vi "Test SCOPE API.vi"() -> ()   [LabVIEW 2021, in "SCOPE.lvlib"]
doc: "SCOPE API Tester.\n\n<b>Note:</b> This VI was modified by the <b>Validate DQMH Module</b> tool to add the 'Show Main VI Diagram on Init' functionality included in DQMH 6.1.\n\n<b>Note:</b> This VI was modified by the <b>Validate DQMH Module</b> tool to upgrade its Error Reported event frame to use an improved mechanism for displaying error information.\n\n<b>Note:</b> This VI was modified by the <b>Validate DQMH Module</b> tool to remove code to stop the main loop on error, and instead display the most recent error on the tester front panel."
uses:
  SCOPE.lvlib
  <vilib>/Utility/error.llb/DialogType.ctl
panel:
  in  "UnLoad in SubPane":bool
  in  "Load in SubPane":bool
  out "last error":errorcluster
  in  "Show Main VI Diagram on Init (F)":bool
  in  "AcqTime":dbl=20.0
  in  "Acquire Signal":bool
  out "ModuleName":string
  in  "Sim?":bool
  in  "Simulation":bool
  in  "Show Block Diagram":bool
  in  "Stop Module":bool
  in  "Start Module":bool
  in  "Hide Module Panel":bool
  in  "Show Module Panel":bool
  out "Status":string
  out "Module Running?":bool
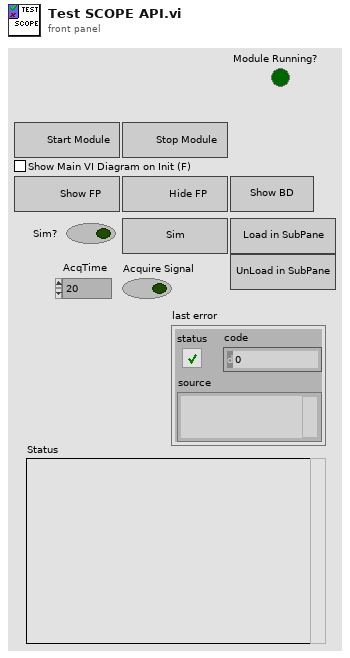
[diagram p1: front panel]
types:
  T1 = typedef "SCOPE.lvlib/Broadcast Events--cluster.ctl" = cluster{"Module Did Init":refnum<user-event>, "Status Updated":refnum<user-event>, "Error Reported":refnum<user-event>, "Module Did Stop":refnum<user-event>, "Update Module Execution Status":refnum<user-event>}
  T2 = typedef "DialogType.ctl" = u16
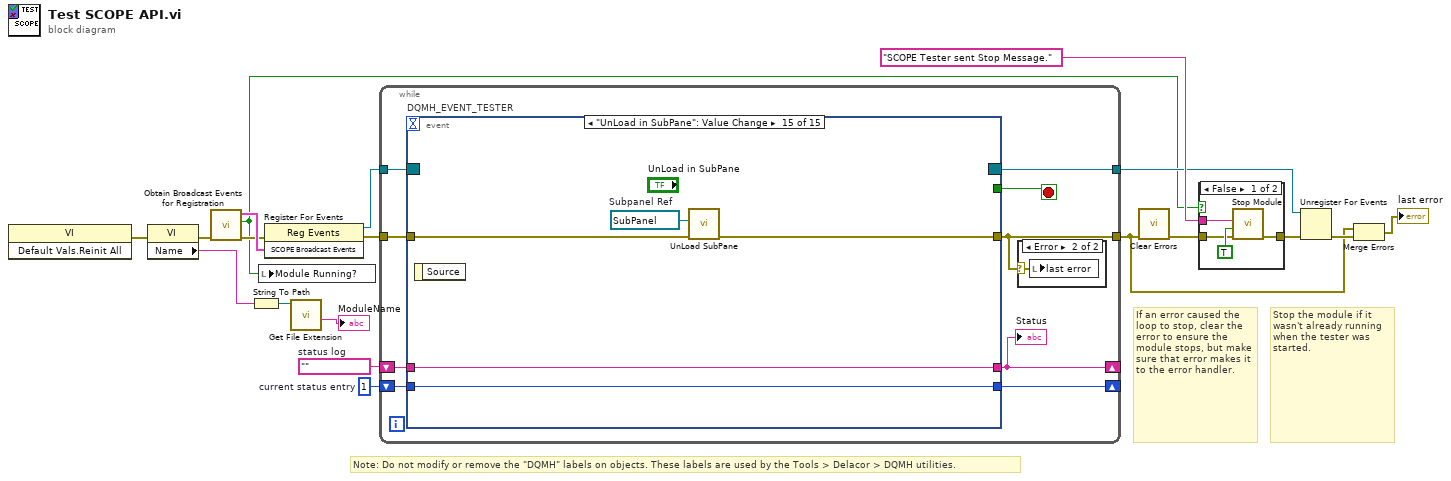
[diagram p0: block diagram]
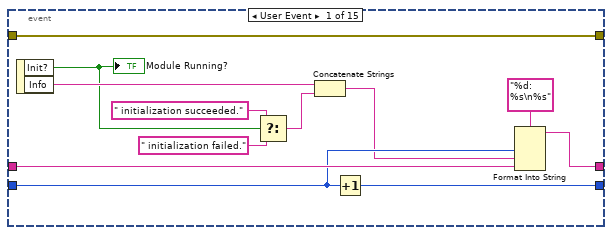
[diagram p4: hidden frame]
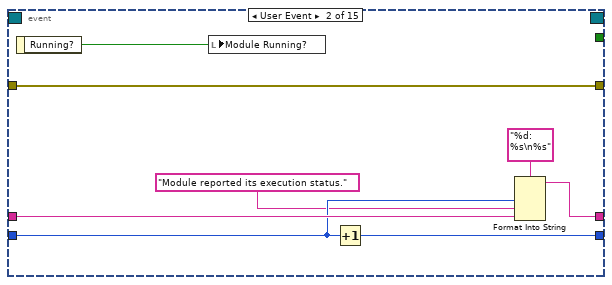
[diagram p5: hidden frame]
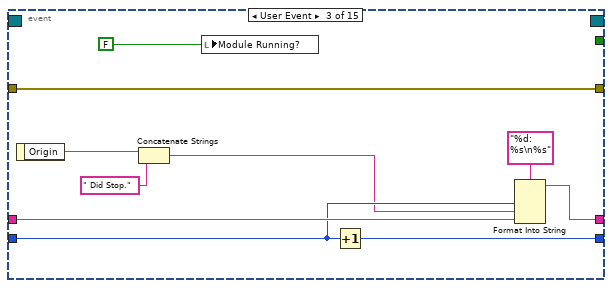
[diagram p6: hidden frame]
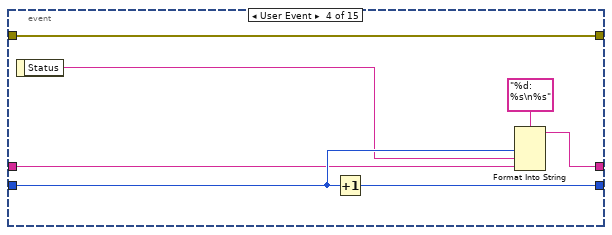
[diagram p7: hidden frame]
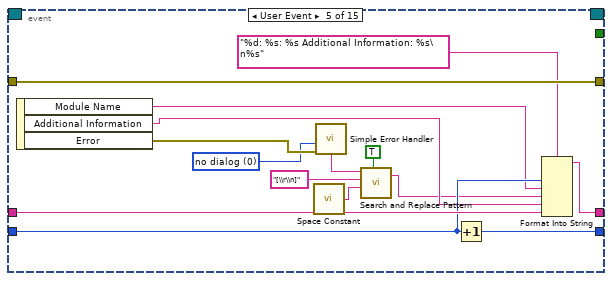
[diagram p8: hidden frame]
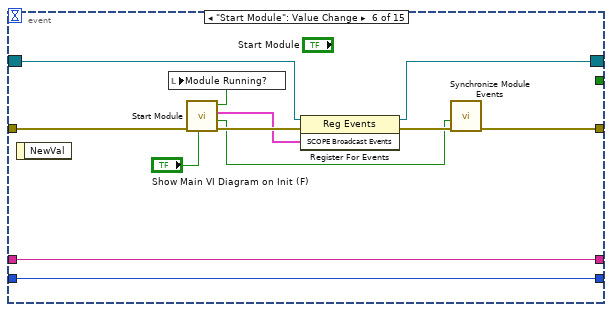
[diagram p9: hidden frame]
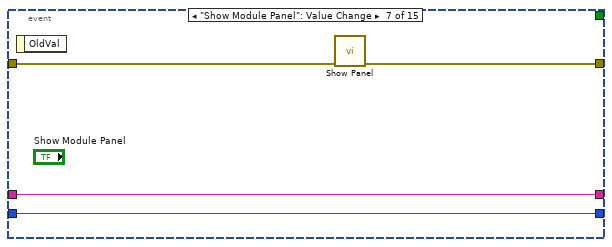
[diagram p10: hidden frame]
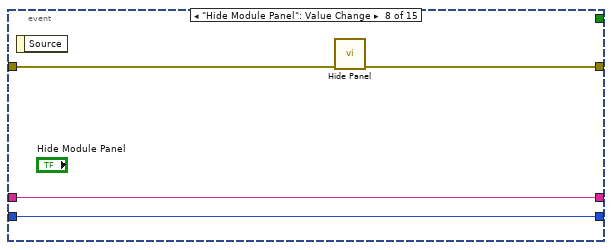
[diagram p11: hidden frame]
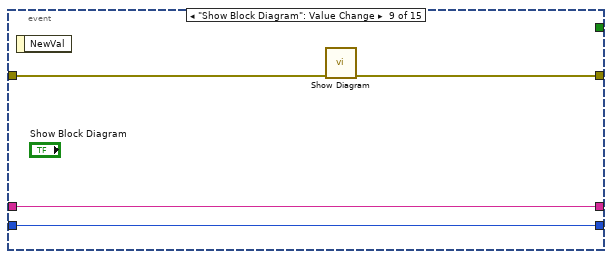
[diagram p12: hidden frame]
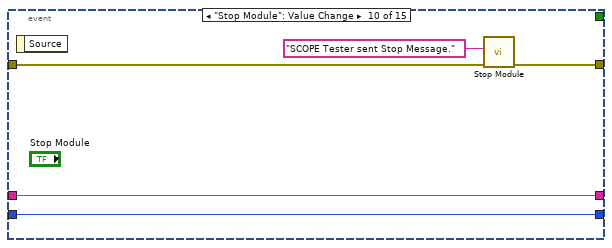
[diagram p13: hidden frame]
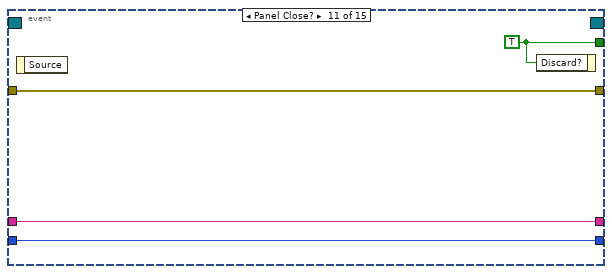
[diagram p14: hidden frame]
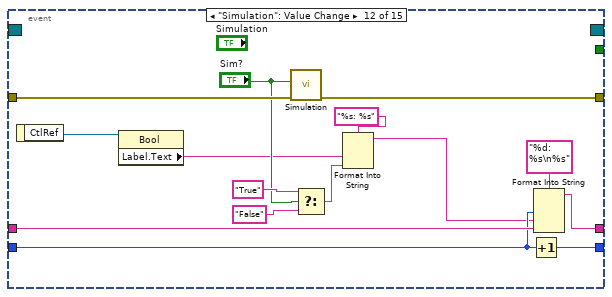
[diagram p15: hidden frame]
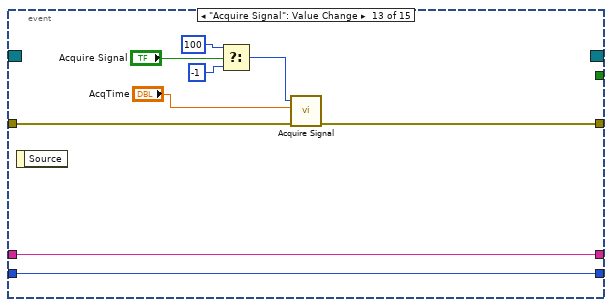
[diagram p16: hidden frame]
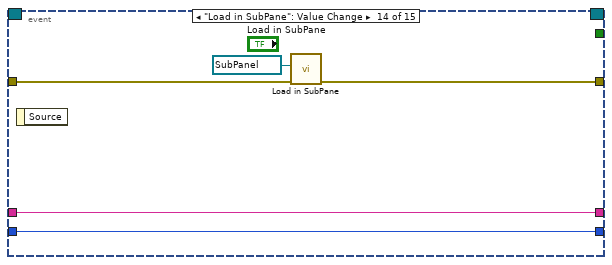
[diagram p17: hidden frame]
diagram:
  w15 = 1  # current status entry
  w16 = ""  # status log
  # "Stop the module if it wasn't already running when the tester was started."
  # "If an error caused the loop to stop, clear the error to ensure the module stops, but make sure that error makes it to the error handler."
  # "Note: Do not modify or remove the \"DQMH\" labels on objects. These labels are used by the Tools > Delacor > DQMH utilities."
  n1 = invoke on="Invoke Node" class="VI" method="Default Vals.Reinit All"() -> (error out=w6:errorcluster)  [unwired: 3 in, 2 out]
  n2 = property on="Property Node" class="VI"(error in=w6) -> (error out=w5:errorcluster, "Name"=w3:string)  [unwired: 1 in, 1 out]
  n3 = call "Obtain Broadcast Events for Registration.vi"("error in (no error)"=w5) -> ("error out"=w8:errorcluster, "Already running?"=w7:bool, "SCOPE Broadcast Events"=w13:T1)  [unwired: 8 in]
  n4 = String To Path(string=w3) -> (path=w2:path)
  n5 = local write "Module Running?"(w7) -> ()
  n6 = register-events(error in=w8, w13) -> (reference out=w12:refnum<event-registration>, error out=w14:errorcluster)  [unwired: 1 in]
  n7 = call <vilib>:"Get File Extension.vi"("file"=w2) -> ("filename without extension"=→"ModuleName":string)  [unwired: 6 in, 4 out]
  n8 = while {
    tunnel: w12 -> [w28]
    tunnel: [w21] -> w9
    shift-right: [w24] -> _
    shift-left: w16 -> [w26]
    shift-right: [w25] -> _
    shift-left: w15 -> [w27]
    tunnel: w14 -> [w23]
    tunnel: [w22] -> w11
    stop <- w20 stop-if-true
    n9 = event "DQMH_EVENT_TESTER" shown="[14] \"UnLoad in SubPane\": Value Change" {
      selector: w28 -> [_ _ _ _ _ w87 _ _ _ _ _ _ _ _ _]
      dyn-events: [_ _ _ _ _ w86 _ _ _ _ _ _ _ _ _] -> w22
      timeout: _ -> [_ _ _ _ _ _ _ _ _ _ _ _ _ _ _]
      tunnel: [_ _ _ _ _ _ _ _ _ _ w114 _ _ _ _] -> w20
      tunnel: [w41 w43 w50 w60 w81 w85 w97 w101 w102 w108 w111 w128 w135 w140 w145] -> w21
      tunnel: w27 -> [w38 w47 w57 w63 w78 w90 w95 w99 w103 w109 w112 w123 w136 w141 w146]
      tunnel: w26 -> [w39 w48 w58 w62 w80 w91 w96 w100 w104 w110 w113 w126 w137 w142 w147]
      tunnel: [w36 w45 w55 w64 w79 w91 w96 w100 w104 w110 w113 w125 w137 w142 w147] -> w24
      tunnel: [w37 w46 w56 w66 w77 w90 w95 w99 w103 w109 w112 w124 w136 w141 w146] -> w25
      tunnel: w23 -> [w41 w43 w50 w60 w81 w84 w94 w98 w105 w106 w111 w129 w138 w143 w148]
      event User Event {
        n10 = event-data() -> ("Init?"=w33:bool, "Info"=w35:string)  [unwired: 1 in]
        "Module Running?" <- w33
        n11 = Select(t=" initialization succeeded.", s=w33, f=" initialization failed.") -> (s? t:f=w30:string)
        n12 = Concatenate Strings(w35, w30) -> (w34:string)
        n13 = Increment(x=w38) -> (x+1=w37:i32)
        n14 = Format Into String(format string="%d: %s\n%s", w38, w34, w39) -> (resulting string=w36:string)  [unwired: 2 in, 1 out]
      }
      event User Event {
        n15 = event-data() -> ("Running?"=w42:bool)  [unwired: 1 in]
        n16 = local write "Module Running?"(w42) -> ()
        n17 = Increment(x=w47) -> (x+1=w46:i32)
        n18 = Format Into String(format string="%d: %s\n%s", w47, "Module reported its execution status.", w48) -> (resulting string=w45:string)  [unwired: 2 in, 1 out]
      }
      event User Event {
        n19 = event-data() -> ("Origin"=w54:string)  [unwired: 1 in]
        n20 = Concatenate Strings(w54, " Did Stop.") -> (w53:string)
        n21 = local write "Module Running?"(FALSE ("Module Did Init?")) -> ()
        n22 = Increment(x=w57) -> (x+1=w56:i32)
        n23 = Format Into String(format string="%d: %s\n%s", w57, w53, w58) -> (resulting string=w55:string)  [unwired: 2 in, 1 out]
      }
      event User Event {
        n24 = event-data() -> ("Status"=w61:string)  [unwired: 1 in]
        n25 = Increment(x=w63) -> (x+1=w66:i32)
        n26 = Format Into String(format string="%d: %s\n%s", w63, w61, w62) -> (resulting string=w64:string)  [unwired: 2 in, 1 out]
      }
      event User Event {
        w73 = T2 0 items=["no dialog", "OK message", "continue or stop message", "OK message + warnings", "continue/stop + warnings"] ("type of dialog (OK msg:1)")
        n27 = event-data() -> ("Module Name"=w74:string, "Additional Information"=w75:string, "Error"=w76:errorcluster)  [unwired: 1 in]
        n28 = call <vilib>:"Space Constant.vi"() -> ("String"=w69:string)
        n29 = call <vilib>:"Simple Error Handler.vi"("type of dialog (OK msg:1)"=w73, "error in (no error)"=w76) -> ("message"=w72:string)  [unwired: 3 in, 4 out]
        n30 = call <vilib>:"Search and Replace Pattern.vi"("string"=w72, "regular expression (\"\")"="[\\r\\n]" ("regular expression (\"\")"), "replace string (\"\")"=w69, "replace all? (F)"=TRUE ("replace all CR/LF with spaces")) -> ("result string"=w71:string)  [unwired: 1 in, 1 out]
        n31 = Increment(x=w78) -> (x+1=w77:i32)
        n32 = Format Into String(format string="%d: %s: %s Additional Information: %s\n%s", w78, w74, w71, w75, w80) -> (resulting string=w79:string)  [unwired: 2 in, 1 out]
      }
      event "Start Module": Value Change {
        n33 = event-data() -> ()  [unwired: 1 in, 1 out]
        n34 = call "Start Module.vi"("Show Main VI Diagram on Init (F)"="Show Main VI Diagram on Init (F)", "error in (no error)"=w84) -> ("error out"=w92:errorcluster, "Wait for Event Sync?"=w89:bool, "SCOPE Broadcast Events"=w88:T1, "Module Was Already Running?"=w83:bool)  [unwired: 5 in, 1 out]
        n35 = local write "Module Running?"(w83) -> ()
        n36 = register-events(reference=w87, error in=w92, w88) -> (reference out=w86:refnum<event-registration>, error out=w93:errorcluster)
        n37 = call "Synchronize Module Events.vi"("error in (no error)"=w93, "Wait for Event Sync?"=w89) -> ("error out"=w85:errorcluster)  [unwired: 9 in]
      }
      event "Show Module Panel": Value Change {
        n38 = event-data() -> ()  [unwired: 1 in, 1 out]
        n39 = call "Show Panel.vi"("error in (no error)"=w94) -> ("error out"=w97:errorcluster)  [unwired: 10 in]
      }
      event "Hide Module Panel": Value Change {
        n40 = event-data() -> ()  [unwired: 1 in, 1 out]
        n41 = call "Hide Panel.vi"("error in (no error)"=w98) -> ("error out"=w101:errorcluster)  [unwired: 10 in]
      }
      event "Show Block Diagram": Value Change {
        n42 = event-data() -> ()  [unwired: 1 in, 1 out]
        n43 = call "Show Diagram.vi"("error in (no error)"=w105) -> ("error out"=w102:errorcluster)  [unwired: 10 in]
      }
      event "Stop Module": Value Change {
        n44 = event-data() -> ()  [unwired: 1 in, 1 out]
        n45 = call "Stop Module.vi"("error in (no error)"=w106, "Origin"="SCOPE Tester sent Stop Message.") -> ("error out"=w108:errorcluster)  [unwired: 9 in]
      }
      event Panel Close? {
        w114 = TRUE ("Discard?")
        n46 = event-data() -> ()  [unwired: 1 in, 1 out]
        n47 = event-data ("Event Filter Node")("Discard?"=w114) -> ()  [unwired: 1 in, 1 out]
      }
      event "Simulation": Value Change {
        n48 = event-data() -> ("CtlRef"=w122:refnum<vi>)  [unwired: 1 in]
        n49 = property on="Property Node" class="Bool"(reference=w122) -> ("Label.Text"=w117:string)  [unwired: 1 in, 2 out]
        n50 = call "Simulation.vi"("error in (no error)"=w129, "Sim?"="Sim?") -> ("error out"=w128:errorcluster)  [unwired: 9 in]
        n51 = Select(t="True", s="Sim?", f="False") -> (s? t:f=w119:string)
        n52 = Format Into String(format string="%s: %s", w117, w119) -> (resulting string=w116:string)  [unwired: 2 in, 1 out]
        n53 = Increment(x=w123) -> (x+1=w124:i32)
        n54 = Format Into String(format string="%d: %s\n%s", w123, w116, w126) -> (resulting string=w125:string)  [unwired: 2 in, 1 out]
      }
      event "Acquire Signal": Value Change {
        n55 = event-data() -> ()  [unwired: 1 in, 1 out]
        n56 = Select(t=100, s="Acquire Signal", f=-1) -> (s? t:f=w132:i32)
        n57 = call "Acquire Signal.vi"("error in"=w138, "AcqTime"="AcqTime", "Rate"=w132) -> ("error out"=w135:errorcluster)  [unwired: 8 in]
      }
      event "Load in SubPane": Value Change {
        n58 = event-data() -> ()  [unwired: 1 in, 1 out]
        n59 = call "Load in SubPane.vi"("error in"=w143, "Subpanel Ref"=refnum<vi> refnum) -> ("error out"=w140:errorcluster)  [unwired: 9 in]
      }
      event "UnLoad in SubPane": Value Change {
        w144 = refnum<vi> refnum  # Subpanel Ref
        n60 = event-data() -> ()  [unwired: 1 in, 1 out]
        n61 = call "UnLoad SubPane.vi"("error in"=w148, "Subpanel Ref"=w144) -> ("error out"=w145:errorcluster)  [unwired: 9 in]
      }
    }
    "Status" <- w24
    n62 = case "DQMH_TESTER_ERROR_LOCAL" shown="Error" w21 {
      selector: w21 -> [_ w29]
      frame No Error {
      }
      frame Error {
        n63 = local write "last error"(w29) -> ()
      }
    }
  }
  n64 = call <vilib>:"Clear Errors.vi"("error in (no error)"=w9) -> ("error out"=w10:errorcluster)  [unwired: 5 in, 1 out]
  n65 = case shown="False" w7 {
    tunnel: [w152 w153] -> w18
    tunnel: "SCOPE Tester sent Stop Message." ("Origin") -> [w151 _]
    tunnel: w10 -> [w149 w153]
    frame False {
      n66 = call "Stop Module.vi"("error in (no error)"=w149, "Wait for Module to Stop? (F)"=TRUE ("Wait for Module to stop?"), "Origin"=w151) -> ("error out"=w152:errorcluster)  [unwired: 8 in]
    }
    frame True {
    }
  }
  n67 = Unregister For Events(event registration refnum=w11, error in=w18) -> (error out=w19:errorcluster)
  n68 = Merge Errors(w9, w19) -> (→"last error":errorcluster)
